vi "treeAddComponent.vi"(8 "error in (no error)":errorcluster, 9 "DisplayType in":T1, 10 "Component in":refnum<class "IComponent.lvclass">, 11 "Tree Ref in":refnum<vi>) -> (0 "error out":errorcluster, 3 "Tree Ref out":refnum<vi>)   [LabVIEW 2022 SP3, in "Property Editor.lvlib"]
uses:
  Property Editor.lvlib
  Public/Classes/IComponent/IComponent.lvclass
  Public/Classes/daqUtils/Tree/Tree.lvlib
  Public/Classes/IBaseObject/IBaseObject.lvclass
  Public/Classes/IComponentStatusContainer/IComponentStatusContainer.lvclass
  Public/Classes/IBaseObject/Polymorphic/borrowInterface/borrowFolderInterface.vi
  Public/Classes/IBaseObject/Polymorphic/borrowInterface/borrowSyncComponentInterface.vi
  Public/Classes/IBaseObject/Polymorphic/borrowInterface/borrowDeviceInterface.vi
  Public/Classes/IBaseObject/Polymorphic/borrowInterface/borrowInputPortInterface.vi
  Public/Classes/IBaseObject/Polymorphic/borrowInterface/borrowFunctionBlockInterface.vi
  Public/Classes/IBaseObject/Polymorphic/borrowInterface/borrowSignalInterface.vi
  Public/Classes/IBaseObject/Polymorphic/borrowInterface/borrowChannelInterface.vi
  TypeDef/DisplayType.ctl
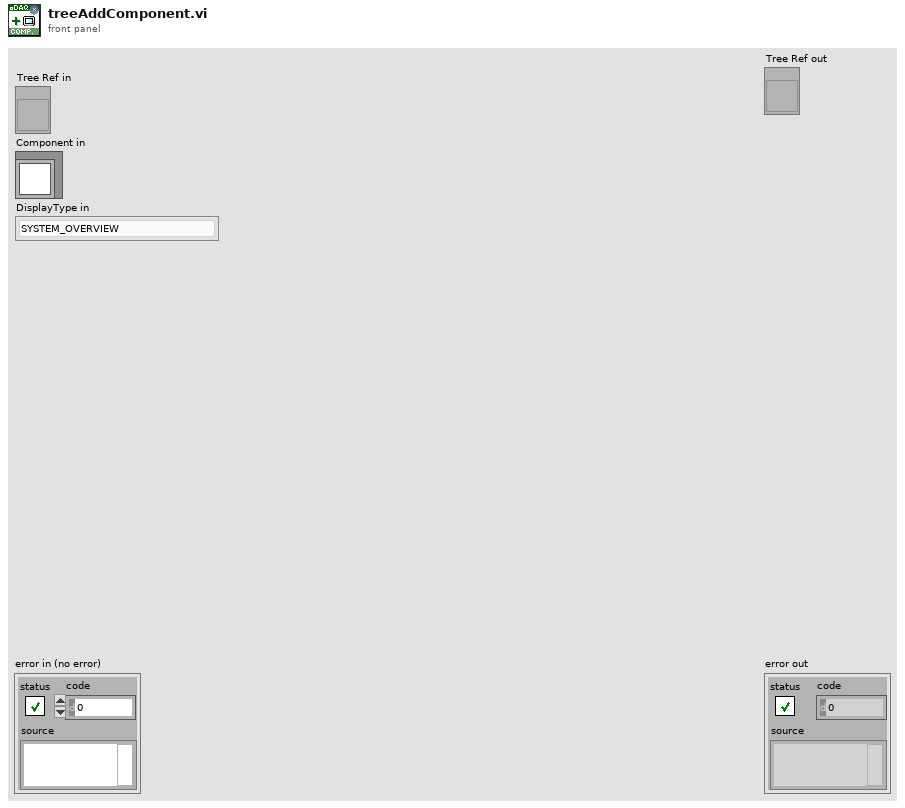
[diagram p1: front panel]
types:
  T1 = typedef "Property Editor.lvlib/DisplayType.ctl" = enum16{"SYSTEM_OVERVIEW", "SIGNALS", "CHANNELS", "FUNCTION_BLOCKS", "TOPOLOGY", "TOPOLOGY_CUSTOM_COMPONENTS", "UNSPECIFIED"}
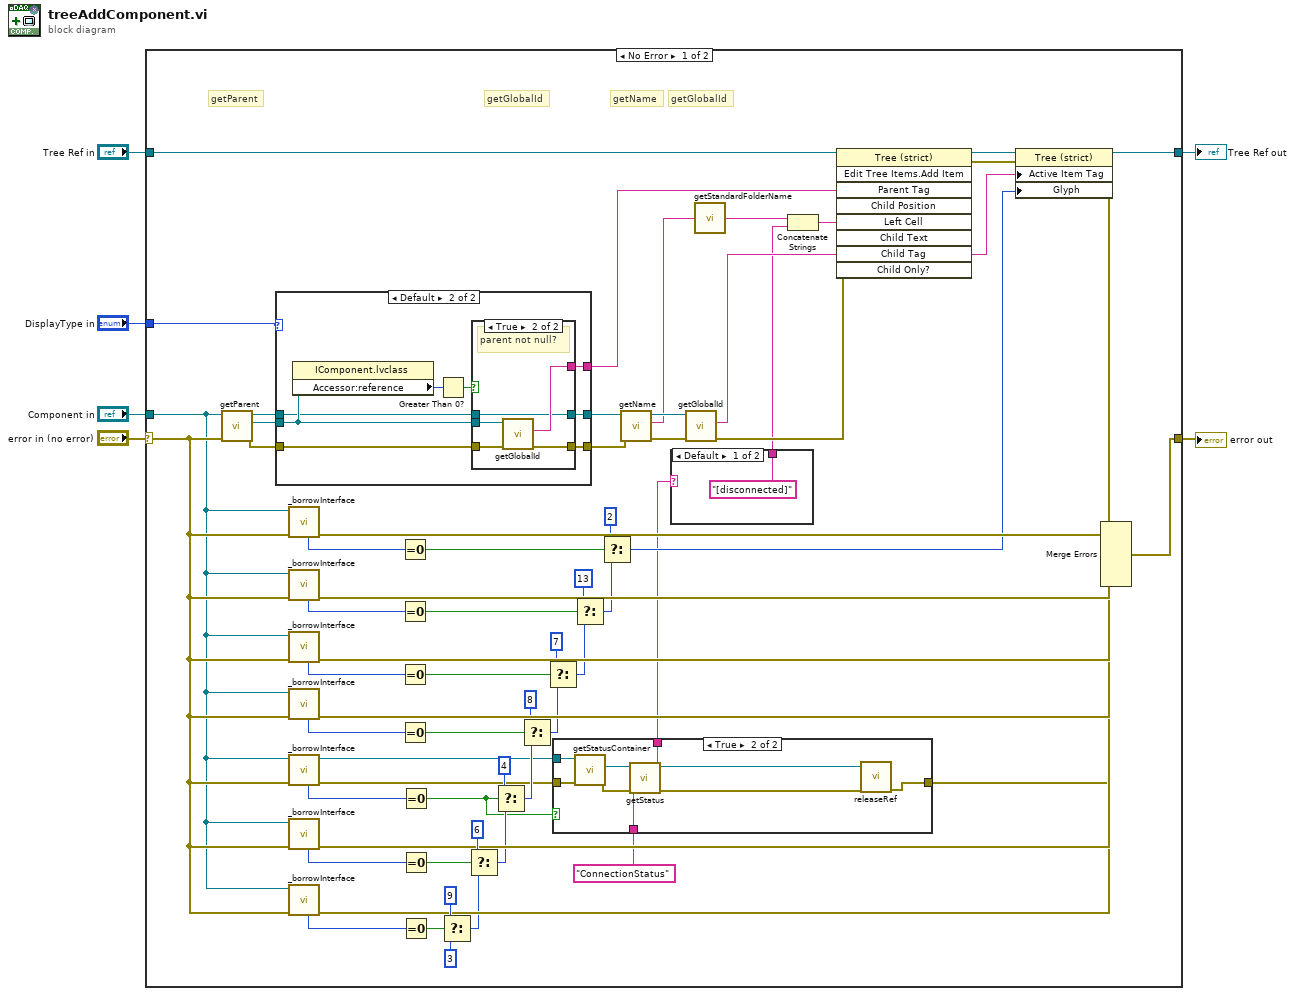
[diagram p0: block diagram]
diagram:
  n1 = case shown="No Error" "error in (no error)" {
    selector: "error in (no error)" -> [w24 w99]
    tunnel: [w10 w99] -> w6
    tunnel: "Tree Ref in" -> [w69 w98]
    tunnel: [w19 w98] -> w3
    tunnel: "Component in" -> [w23 _]
    tunnel: "DisplayType in" -> [w60 _]
    frame No Error {
      # "getGlobalId"
      # "getName"
      # "getGlobalId"
      # "getParent"
      n2 = call "getParent.vi"("error in (no error)"=w24, "IComponent in"=w23) -> ("error out"=w65:errorcluster, "Parent out"=w66:refnum<class "IComponent.lvclass">, "IComponent out"=w64:refnum<class "IComponent.lvclass">)  [unwired: 7 in]
      n3 = case shown="Default" w60 {
        tunnel: [_ w90] -> w59
        tunnel: [w81 w87] -> w63
        tunnel: w66 -> [_ w86]
        tunnel: w65 -> [w82 w85]
        tunnel: [w82 w84] -> w62
        tunnel: w64 -> [w81 w83]
        frame "SIGNALS".."FUNCTION_BLOCKS" {
        }
        frame Default {
          n4 = property class="IComponent.lvclass"(reference=w86) -> ("Accessor:reference"=w89:i64)  [unwired: 1 in, 2 out]
          n5 = Greater Than 0?(x=w89) -> (x > 0?=w88:bool)
          n6 = case shown="True" w88 {
            tunnel: [w91 w93] -> w87
            tunnel: [_ w97] -> w90
            tunnel: w86 -> [_ w96]
            tunnel: w85 -> [w92 w95]
            tunnel: [w92 w94] -> w84
            tunnel: w83 -> [w91 w93]
            frame False {
              # "parent not null?"
            }
            frame True {
              # "parent not null?"
              n7 = call "getGlobalId.vi"("error in (no error)"=w95, "IComponent in"=w96) -> ("error out"=w94:errorcluster, "GlobalId out"=w97:string)  [unwired: 7 in, 1 out]
            }
          }
        }
      }
      n8 = call-poly "_borrowInterface.vi"("error in (no error)"=w24, "IBaseObject in"=w23) -> ("error out"=w56:errorcluster, "err"=w22:u32)  [unwired: 6 in, 2 out]
      n9 = call-poly "_borrowInterface.vi"("error in (no error)"=w24, "IBaseObject in"=w23) -> ("error out"=w55:errorcluster, "err"=w52:u32)  [unwired: 6 in, 2 out]
      n10 = call-poly "_borrowInterface.vi"("error in (no error)"=w24, "IBaseObject in"=w23) -> ("error out"=w54:errorcluster, "err"=w51:u32)  [unwired: 6 in, 2 out]
      n11 = call-poly "_borrowInterface.vi"("error in (no error)"=w24, "IBaseObject in"=w23) -> ("error out"=w53:errorcluster, "err"=w50:u32)  [unwired: 6 in, 2 out]
      n12 = call-poly "_borrowInterface.vi"("error in (no error)"=w24, "IBaseObject in"=w23) -> ("error out"=w13:errorcluster, "IBaseObject out"=w14:refnum<class "IComponent.lvclass">, "err"=w49:u32)  [unwired: 6 in, 1 out]
      n13 = call-poly "_borrowInterface.vi"("error in (no error)"=w24, "IBaseObject in"=w23) -> ("error out"=w29:errorcluster, "err"=w33:u32)  [unwired: 6 in, 2 out]
      n14 = call-poly "_borrowInterface.vi"("error in (no error)"=w24, "IBaseObject in"=w23) -> ("error out"=w28:errorcluster, "err"=w32:u32)  [unwired: 6 in, 2 out]
      n15 = Equal To 0?(x=w22) -> (x = 0?=w48:bool)
      n16 = Equal To 0?(x=w52) -> (x = 0?=w45:bool)
      n17 = Equal To 0?(x=w51) -> (x = 0?=w42:bool)
      n18 = Equal To 0?(x=w50) -> (x = 0?=w39:bool)
      n19 = Equal To 0?(x=w49) -> (x = 0?=w15:bool)
      n20 = Equal To 0?(x=w33) -> (x = 0?=w35:bool)
      n21 = Equal To 0?(x=w32) -> (x = 0?=w30:bool)
      n22 = Select(t=9 ("Child Position"), s=w30, f=3) -> (s? t:f=w26:i32)
      n23 = Select(t=6 ("Child Position"), s=w35, f=w26) -> (s? t:f=w27:i32)
      n24 = Select(t=4 ("Child Position"), s=w15, f=w27) -> (s? t:f=w36:i32)
      n25 = Select(t=8 ("Child Position"), s=w39, f=w36) -> (s? t:f=w38:i32)
      n26 = Select(t=7 ("Child Position"), s=w42, f=w38) -> (s? t:f=w41:i32)
      n27 = case shown="True" w15 {
        tunnel: w14 -> [_ w80]
        tunnel: w13 -> [w71 w79]
        tunnel: [w71 w74] -> w12
        tunnel: "ConnectionStatus" -> [_ w73]
        tunnel: [_ w72] -> w8
        frame False {
        }
        frame True {
          n28 = call "getStatusContainer.vi"("error in (no error)"=w79, "IComponent in"=w80) -> ("error out"=w77:errorcluster, "IComponentStatusContainer out"=w78:refnum<class "IComponentStatusContainer.lvclass">)  [unwired: 7 in, 1 out]
          n29 = call "getStatus.vi"("error in (no error)"=w77, "Status Name in"=w73, "IComponent in"=w78) -> ("error out"=w75:errorcluster, "Status out"=w72:string, "IComponent out"=w76:refnum<class "IComponentStatusContainer.lvclass">)  [unwired: 6 in]
          n30 = call-dynamic "releaseRef.vi"("error in (no error)"=w75, "IBaseObject in"=w76) -> ("error out"=w74:errorcluster)  [unwired: 9 in]
        }
      }
      n31 = Select(t=13 ("Child Position"), s=w45, f=w41) -> (s? t:f=w44:i32)
      n32 = Select(t=2 ("Child Position"), s=w48, f=w44) -> (s? t:f=w16:i32)
      n33 = call "getName.vi"("error in (no error)"=w62, "IComponent in"=w63) -> ("error out"=w68:errorcluster, "Name out"=w58:string, "IComponent out"=w67:refnum<class "IComponent.lvclass">)  [unwired: 7 in]
      n34 = case shown="Default" w8 {
        tunnel: ["[disconnected]" _] -> w7
        frame Default {
        }
        frame "", "Connected" {
        }
      }
      n35 = call "getGlobalId.vi"("error in (no error)"=w68, "IComponent in"=w67) -> ("error out"=w61:errorcluster, "GlobalId out"=w17:string)  [unwired: 7 in, 1 out]
      n36 = call "getStandardFolderName.vi"("Name in"=w58) -> ("Folder name out"=w57:string)  [unwired: 4 in]
      n37 = Concatenate Strings(w57, w7) -> (w9:string)
      n38 = invoke class="Tree (strict)" method="Edit Tree Items.Add Item"(reference=w69, error in=w61, "Parent Tag"=w59, "Left Cell"=w9, "Child Tag"=w17) -> (reference out=w21:refnum<vi>, error out=w20:errorcluster)  [unwired: 4 in, 7 out]
      n39 = property class="Tree (strict)"(reference=w21, error in=w20, "Active Item Tag"=w17, "Glyph"=w16) -> (reference out=w19:refnum<vi>, error out=w18:errorcluster)
      n40 = Merge Errors(w18, w56, w55, w54, w53, w12, w29, w28) -> (w10:errorcluster)
    }
    frame Error {
    }
  }
  "error out" <- w6
  "Tree Ref out" <- w3
